vi "ARC_Comm Relative Path.vi"(5 "Development Relative Path":string="Development Relative", 7 "Run Time relative path":string, 8 "error in (no error)":errorcluster, 9 "Run-Time File Depth":i32, 10 "Development File Depth":i32, 11 "Root Path":path) -> (0 "error out":errorcluster, 3 "Relative Path":path)   [LabVIEW 2016]
doc: "ÎÄ¼þµÄÏà¶ÔÂ·¾¶¡£ÒÀ¾Ý±à¼­»·¾³»¹ÊÇÔËÐÐ»·¾³£¬ÐèÒªÉè¶¨ÎÄ¼þµÄÂ·¾¶¡£´ËviÌá¹©ÔÚ²»Í¬»·¾³ÏÂµÄÂ·¾¶ÉèÖÃ½Ó¿Ú¡£\n\n***ICON-SYMBOL***\nTitle=Common§\nText1=Relative§\nText2=Path§\nText3= §\nBodyC1=12808703§\nBodyC2=16448250§\nTextC1=0§\nTextC2=0§"
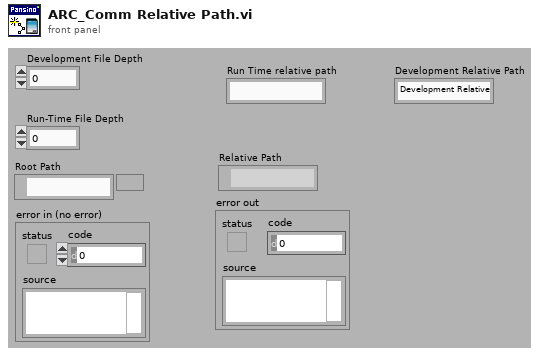
[diagram p1: front panel]
types:
  T1 = enum32{"invalid app kind", "Development System", "Run Time System", "Student Edition", "Embedded LabVIEW", "Evaluation", "Custom"}
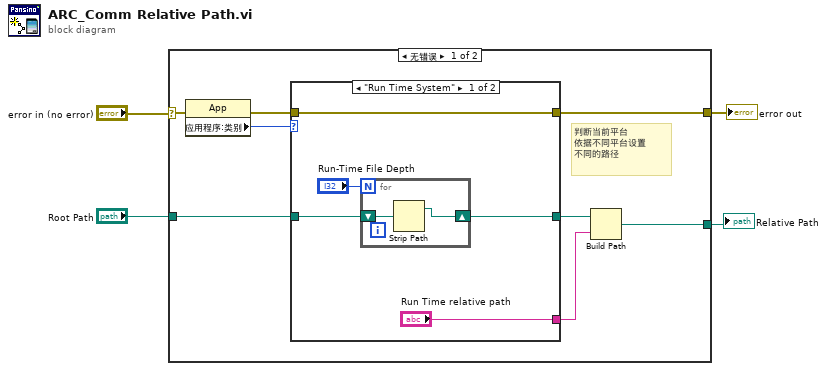
[diagram p0: block diagram]
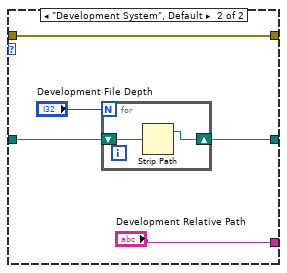
[diagram p2: hidden frame]
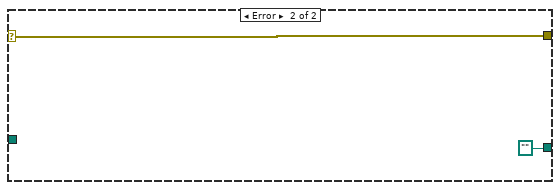
[diagram p3: hidden frame]
diagram:
  n1 = case shown="无错误" "error in (no error)" {
    selector: "error in (no error)" -> [w8 w27]
    tunnel: [w10 path ""] -> w3
    tunnel: [w6 w27] -> w2
    tunnel: "Root Path" -> [w5 _]
    frame No Error {
      # "判断当前平台\n依据不同平台设置\n不同的路径"
      n2 = property class="App"(error in=w8) -> (error out=w7:errorcluster, "应用程序:类别"=w12:T1)  [unwired: 1 in, 1 out]
      n3 = case shown="\"Run Time System\"" w12 {
        tunnel: w5 -> [w17 w24]
        tunnel: [w15 w22] -> w11
        tunnel: ["Run Time relative path" "Development Relative Path"] -> w9
        tunnel: [w13 w20] -> w6
        tunnel: w7 -> [w13 w20]
        frame "Run Time System" {
          n4 = for {
            N: "Run-Time File Depth" -> [_]
            shift-right: [w18] -> w15
            shift-left: w17 -> [w19]
            n5 = Strip Path(path=w19) -> (stripped path=w18:path)  [unwired: 1 out]
          }
        }
        frame "Development System", Default {
          n6 = for {
            N: "Development File Depth" -> [_]
            shift-right: [w25] -> w22
            shift-left: w24 -> [w26]
            n7 = Strip Path(path=w26) -> (stripped path=w25:path)  [unwired: 1 out]
          }
        }
      }
      n8 = Build Path(base path=w11, name or relative path=w9) -> (appended path=w10:path)
    }
    frame Error {
    }
  }
  "Relative Path" <- w3
  "error out" <- w2
